vi "Start Sync.vi"(8 "error in (no error)":errorcluster, 10 "MeasurementPlugin in":refnum<class "MeasurementPluginService.lvclass">, 11 "MeasurementServiceV2 in":refnum<class "MeasurementServiceV2.lvclass">) -> (0 "error out":errorcluster, 3 "MeasurementServiceV2 out":refnum<class "MeasurementServiceV2.lvclass">)   [LabVIEW 2020, in "MeasurementLink Measurement Server.lvlib" / "MeasurementServiceV2.lvclass"]
uses:
  MeasurementServiceV2.lvclass
  MeasurementPluginService/MeasurementPluginService.lvclass
  MeasurementServiceV2.lvclass/MeasurementServiceV2.ctl
  MeasurementLink Measurement Service Base V2/RPC Service/MeasurementService/MeasurementServiceBaseV2.lvclass/MeasurementServiceBaseV2.ctl
  MeasurementLink Measurement Service Base V2/RPC Service/MeasurementService/Accessor/Read Server RPC Methods.vi
  MeasurementLink Measurement Service Base V2/RPC Service/MeasurementService/MeasurementServiceBaseV2.lvclass
  C:/Program Files/National Instruments/LabVIEW 2020/vi.lib/gRPC/LabVIEW gRPC Servicer/ServiceBase/ServiceBase.lvclass
  IMeasurementService/IMeasurementService.lvclass
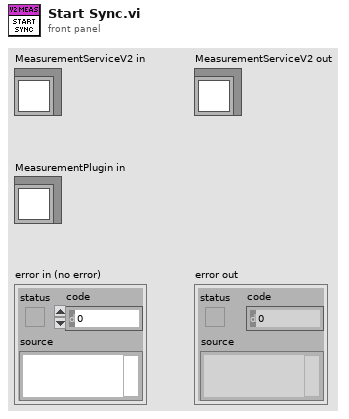
[diagram p1: front panel]
types:
  T1 = typedef "MeasurementLink Measurement Service Base V2.lvlib/MeasurementServiceBaseV2.lvclass/Server gRPC UEs.ctl" = cluster{"MeasurementService GetMetadata gRPC UE":refnum<user-event>, "MeasurementService Measure gRPC UE":refnum<user-event>}
  T2 = typedef "grpc-lvsupport-release.lvlib/grpcId.ctl" = u64
  T3 = typedef "MeasurementLink Measurement Server.lvlib/GetMetadataResponse.ctl" = cluster{"measurement_details":T4, "measurement_signature":T5, "user_interface_details":T11[]}
  T4 = typedef "MeasurementLink Measurement Server.lvlib/MeasurementDetails.ctl" = cluster{"display_name":string, "version":string}
  T5 = typedef "MeasurementLink Measurement Server.lvlib/MeasurementSignature.ctl" = cluster{"configuration_parameters_message_type":string, "configuration_parameters":T6[], "configuration_defaults":T8, "outputs_message_type":string, "outputs":T9[]}
  T6 = typedef "MeasurementLink Measurement Server.lvlib/ConfigurationParameter.ctl" = cluster{"field_number":i32, "type":i32, "name":string, "repeated":bool, "annotations":T7[]}
  T7 = typedef "MeasurementLink Measurement Server.lvlib/ConfigurationParameter_AnnotationsEntry.ctl" = cluster{"key":string, "value":string}
  T8 = typedef "grpc-lvsupport-release.lvlib/Any.ctl" = cluster{"Type Url":string, "Bytes":u8[]}
  T9 = typedef "MeasurementLink Measurement Server.lvlib/Output.ctl" = cluster{"field_number":i32, "type":i32, "name":string, "repeated":bool, "annotations":T10[]}
  T10 = typedef "MeasurementLink Measurement Service Base V2.lvlib/ni_measurementlink_measurement_v2_Output_AnnotationsEntry.ctl" = cluster{"key":string, "value":string}
  T11 = typedef "MeasurementLink Measurement Server.lvlib/UserInterfaceDetails.ctl" = cluster{"file_url":string}
  T12 = typedef "MeasurementLink Measurement Service Base V2.lvlib/ni_measurementlink_measurement_v2_MeasureRequest.ctl" = cluster{"configuration_parameters":T13, "pin_map_context":T14}
  T13 = typedef "MeasurementLink Measurement Service Base V2.lvlib/google_protobuf_Any.ctl" = cluster{"type_url":string, "value":u8[]}
  T14 = typedef "MeasurementLink Measurement Service Base V2.lvlib/ni_measurementlink_PinMapContext.ctl" = cluster{"pin_map_id":string, "sites":i32[]}
  T15 = typedef "MeasurementLink Measurement Server.lvlib/MeasureResponse.ctl" = cluster{"outputs":T16}
  T16 = typedef "MeasurementLink Measurement Server Internal.lvlib/google_protobuf_Any.ctl" = cluster{"type_url":string, "value":u8[]}
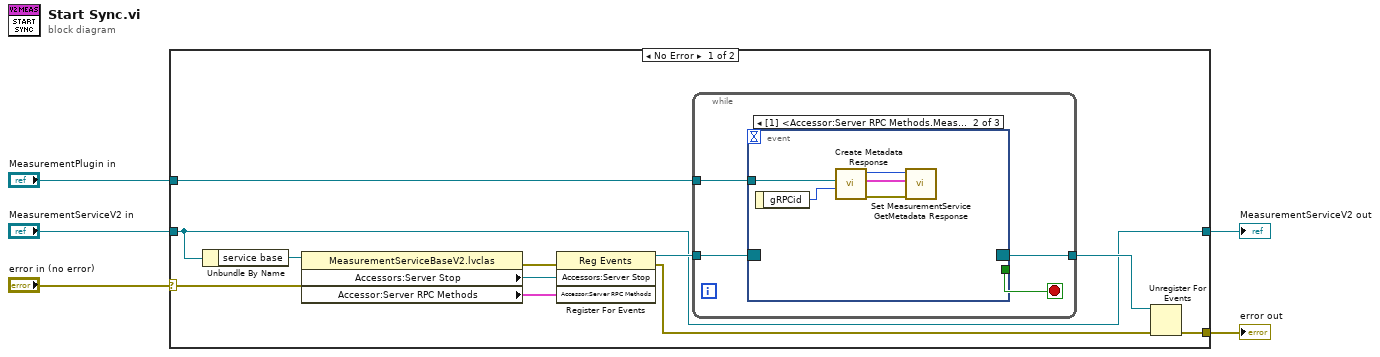
[diagram p0: block diagram]
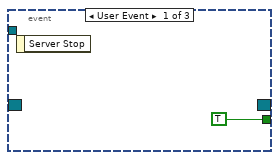
[diagram p2: hidden frame]
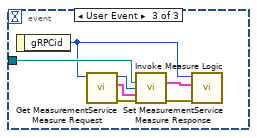
[diagram p3: hidden frame]
diagram:
  n1 = case shown="No Error" "error in (no error)" {
    selector: "error in (no error)" -> [w10 w35]
    tunnel: [w14 w35] -> w3
    tunnel: "MeasurementPlugin in" -> [w11 _]
    tunnel: "MeasurementServiceV2 in" -> [w7 w34]
    tunnel: [w7 w34] -> w1
    frame No Error {
      n2 = Unbundle By Name(w7) -> ("service base"=w13:refnum<class "MeasurementServiceBaseV2.lvclass">)
      n3 = property class="MeasurementServiceBaseV2.lvclas"(reference=w13, error in=w10) -> (error out=w9:errorcluster, "Accessors:Server Stop"=w12:refnum<user-event>, "Accessor:Server RPC Methods"=w8:T1)  [unwired: 1 out]
      n4 = register-events(error in=w9, w12, w8) -> (reference out=w16:refnum<event-registration>, error out=w6:errorcluster)  [unwired: 1 in]
      n5 = while {
        tunnel: w16 -> [w20]
        tunnel: [w19] -> w15
        tunnel: w11 -> [w18]
        stop <- w17 stop-if-true
        n6 = event "RPC Methods Event Structure" shown="[1] <Accessor:Server RPC Methods.MeasurementService GetMetadata gRPC UE>: User Event" {
          selector: w20 -> [_ _ _]
          dyn-events: [_ _ _] -> w19
          timeout: _ -> [_ _ _]
          tunnel: [TRUE _ _] -> w17
          tunnel: w18 -> [_ w23 w32]
          event User Event {
            n7 = event-data() -> ()  [unwired: 1 in, 1 out]
          }
          event User Event {
            n8 = event-data() -> ("gRPCid"=w24:T2)  [unwired: 1 in]
            n9 = call "Create Metadata Response.vi"("gRPCid"=w24, "MeasurementPluginService in"=w23) -> ("error out"=w26:errorcluster, "Get Metadata Response"=w22:T3, "gRPCid out"=w25:T2)  [unwired: 7 in]
            n10 = call "Set MeasurementService GetMetadata Response.vi"("error in (no error)"=w26, "Message Data"=w22, "gRPCid in"=w25) -> ()  [unwired: 8 in, 1 out]
          }
          event User Event {
            n11 = event-data() -> ("gRPCid"=w29:T2)  [unwired: 1 in]
            n12 = call "Get MeasurementService Measure Request.vi"("gRPCid in"=w29) -> ("error out"=w30:errorcluster, "Message Data"=w27:T12, "gRPCid out"=w28:T2)  [unwired: 8 in]
            n13 = call "Invoke Measure Logic.vi"("MeasurementPlugin in"=w32, "gRPCid in"=w28, "MeasureRequest"=w27, "error in (no error)"=w30) -> ("Measure Response"=w31:T15, "error out"=w33:errorcluster)  [unwired: 10 in]
            n14 = call "Set MeasurementService Measure Response.vi"("error in (no error)"=w33, "Message Data"=w31, "gRPCid in"=w29) -> ()  [unwired: 8 in, 1 out]
          }
        }
      }
      n15 = Unregister For Events(event registration refnum=w15, error in=w6) -> (error out=w14:errorcluster)
    }
    frame Error {
    }
  }
  "error out" <- w3
  "MeasurementServiceV2 out" <- w1
